vi "Get Config File or Folder Path.vi"(8 "Error In":errorcluster, 11 "Which file or folder?":T1) -> (0 "Error Out":errorcluster, 1 "File/Folder name string":string, 3 "File Path":path)   [LabVIEW 2020]
doc: "Get the path to the Settings XML file. This is done using the Application Directory function. For more information on how Application Directory calculates its path, right-click the function and choose Help."
uses:
  Typedefs/Which path.ctl
  Global Variables/General Globals.vi
  User Interface/User profiles code/Globals/gl_UsrProfiles globals.vi
  Calibration/Globals/gl_Calibration globals.vi
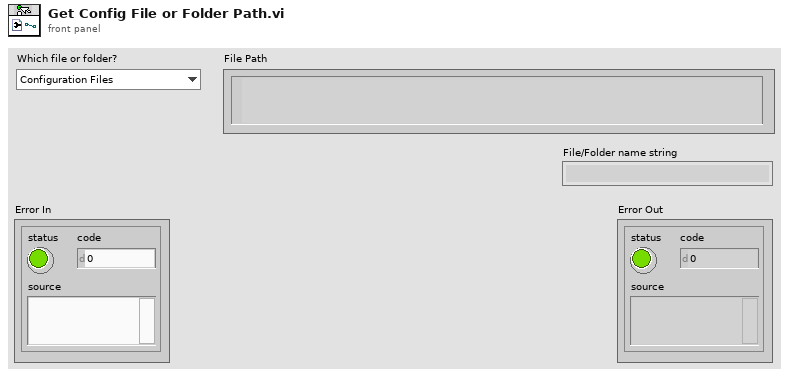
[diagram p1: front panel]
types:
  T1 = typedef "Which path.ctl" = enum16{"Configuration Files", "Calibration Files", "Images", "Setup.ini", "Loaded User profile.ini", "User's-Previous session.ini", "New user profile.ini", "Selected User profile.ini", "User profiles folder", "Power meter scaling.txt", "FOV Cal.ini", "Calibration.ini"}
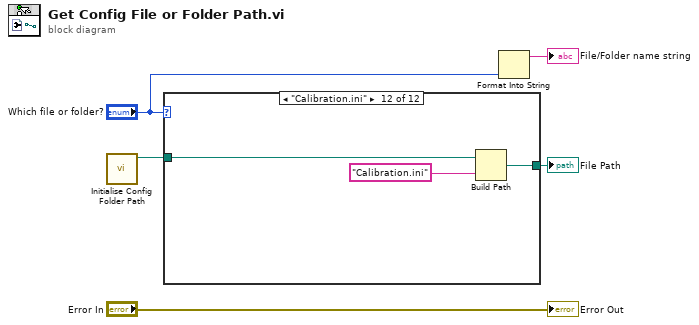
[diagram p0: block diagram]
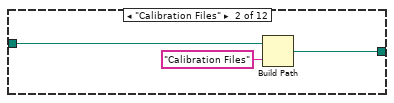
[diagram p3: hidden frame]
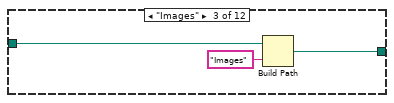
[diagram p4: hidden frame]
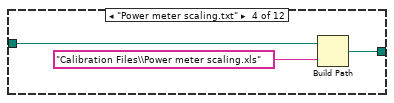
[diagram p5: hidden frame]
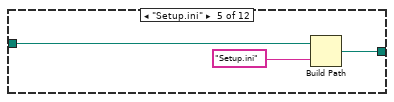
[diagram p6: hidden frame]
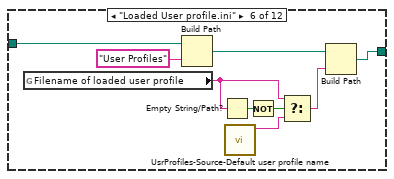
[diagram p7: hidden frame]
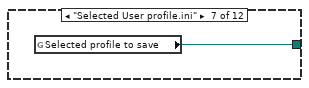
[diagram p8: hidden frame]
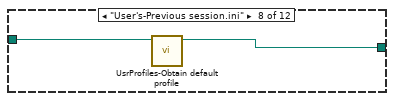
[diagram p9: hidden frame]
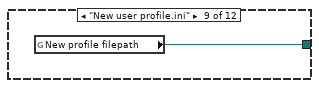
[diagram p10: hidden frame]
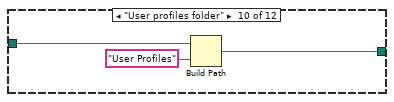
[diagram p11: hidden frame]
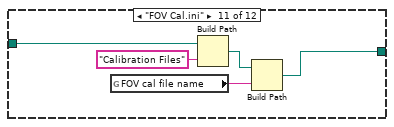
[diagram p12: hidden frame]
diagram:
  n1 = call "Initialise Config Folder Path.vi"() -> ("Config Files Folder Path"=w3:path)  [unwired: 9 in, 2 out]
  n2 = case shown="\"Calibration.ini\"" "Which file or folder?" {
    tunnel: w3 -> [w6 w8 w11 w14 w18 w27 _ w30 _ w34 w36 w41]
    tunnel: [w6 w7 w10 w13 w17 w24 w28 w29 w31 w32 w39 w40] -> w4
    frame "Configuration Files", Default {
    }
    frame "Calibration Files" {
      n3 = Build Path(base path=w8, name or relative path="Calibration Files") -> (appended path=w7:path)
    }
    frame "Images" {
      n4 = Build Path(base path=w11, name or relative path="Images") -> (appended path=w10:path)
    }
    frame "Power meter scaling.txt" {
      n5 = Build Path(base path=w14, name or relative path="Calibration Files\\Power meter scaling.xls") -> (appended path=w13:path)
    }
    frame "Setup.ini" {
      n6 = Build Path(base path=w18, name or relative path="Setup.ini") -> (appended path=w17:path)
    }
    frame "Loaded User profile.ini" {
      n7 = global read "General Globals.vi" "Filename of loaded user profile"() -> (w21:string)
      n8 = Build Path(base path=w27, name or relative path="User Profiles") -> (appended path=w25:path)
      n9 = Empty String/Path?(string/path=w21) -> (empty?=w23:bool)
      n10 = call "UsrProfiles-Source-Default user profile name.vi"() -> ("Default user's profile file name & extension"=w19:string)  [unwired: 11 in]
      n11 = Not(x=w23) -> (.not. x?=w22:bool)
      n12 = Select(t=w21, s=w22, f=w19) -> (s? t:f=w20:string)
      n13 = Build Path(base path=w25, name or relative path=w20) -> (appended path=w24:path)
    }
    frame "Selected User profile.ini" {
      n14 = global read "gl_UsrProfiles globals.vi" "Selected profile to save"() -> (w28:path)
    }
    frame "User's-Previous session.ini" {
      n15 = call "UsrProfiles-Obtain default profile.vi"("Config Files Folder Path"=w30) -> ("\"Default user\" or \"Previous session\" profile's filepath"=w29:path)  [unwired: 10 in]
    }
    frame "New user profile.ini" {
      n16 = global read "gl_UsrProfiles globals.vi" "New profile filepath"() -> (w31:path)
    }
    frame "User profiles folder" {
      n17 = Build Path(base path=w34, name or relative path="User Profiles") -> (appended path=w32:path)
    }
    frame "FOV Cal.ini" {
      n18 = global read "gl_Calibration globals.vi" "FOV cal file name"() -> (w38:string)
      n19 = Build Path(base path=w36, name or relative path="Calibration Files") -> (appended path=w35:path)
      n20 = Build Path(base path=w35, name or relative path=w38) -> (appended path=w39:path)
    }
    frame "Calibration.ini" {
      n21 = Build Path(base path=w41, name or relative path="Calibration.ini") -> (appended path=w40:path)
    }
  }
  "File Path" <- w4
  n22 = Format Into String("Which file or folder?") -> (resulting string=→"File/Folder name string":string)  [unwired: 3 in, 1 out]
  "Error Out" <- "Error In"
